vi "dis_on_test.vi"() -> ()   [LabVIEW 2011]
panel:
  in  "milliseconds to wait":u32=20
  in  "Starting Voltage":dbl=0.4
  in  "Goal Signal":dbl=1.0
  out "Generator Voltage 2":string
  out "Over 2":bool
  out "Signal 2":dbl
  out "Signal":dbl
  out "Over":bool
  out "Generator Voltage":string
  out "Read Back":string
  out "Check":string
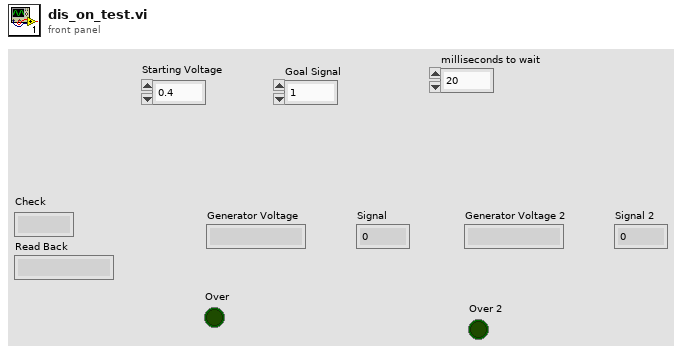
[diagram p1: front panel]
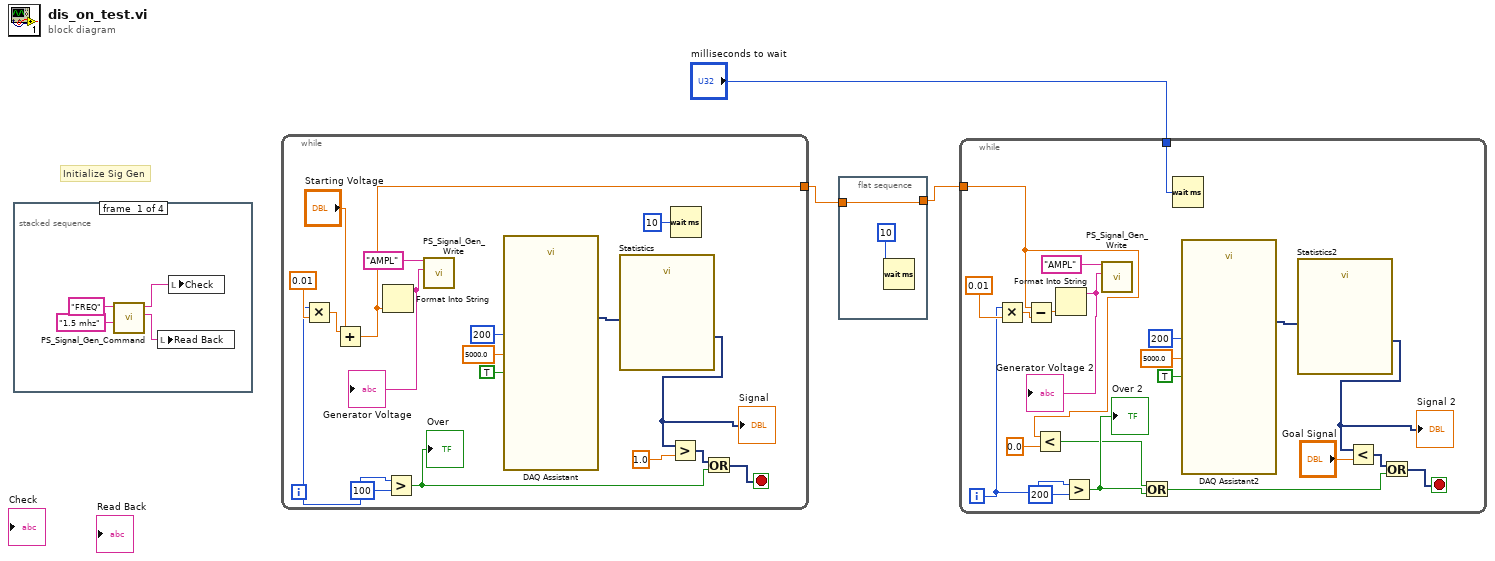
[diagram p0: block diagram]
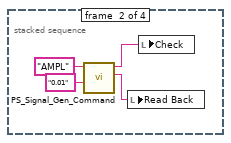
[diagram p2: hidden frame]
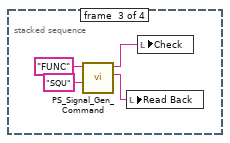
[diagram p3: hidden frame]
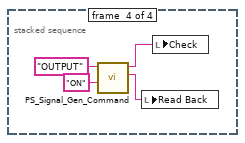
[diagram p4: hidden frame]
diagram:
  # "Initialize Sig Gen"
  n1 = stacked-sequence {
    frame #0 {
      n2 = call "PS_Signal_Gen_Command.vi"("Value String"="1.5 mhz", "Command String"="FREQ") -> ("Read Back"=w4:string, "Request String"=w5:string)  [unwired: 7 in, 1 out]
      n3 = local write "Read Back"(w4) -> ()
      n4 = local write "Check"(w5) -> ()
    }
    frame #1 {
      n5 = call "PS_Signal_Gen_Command.vi"("Value String"="0.01", "Command String"="AMPL") -> ("Read Back"=w8:string, "Request String"=w9:string)  [unwired: 7 in, 1 out]
      n6 = local write "Read Back"(w8) -> ()
      n7 = local write "Check"(w9) -> ()
    }
    frame #2 {
      n8 = call "PS_Signal_Gen_Command.vi"("Value String"="SQU", "Command String"="FUNC") -> ("Read Back"=w12:string, "Request String"=w13:string)  [unwired: 7 in, 1 out]
      n9 = local write "Read Back"(w12) -> ()
      n10 = local write "Check"(w13) -> ()
    }
    frame #3 {
      n11 = call "PS_Signal_Gen_Command.vi"("Value String"="ON", "Command String"="OUTPUT") -> ("Read Back"=w16:string, "Request String"=w17:string)  [unwired: 7 in, 1 out]
      n12 = local write "Read Back"(w16) -> ()
      n13 = local write "Check"(w17) -> ()
    }
  }
  n14 = while {
    tunnel: [w23] -> w3
    i -> [w36]
    stop <- w30 stop-if-true
    n15 = Multiply(x=w36, y=0.01) -> (x*y=w22:dbl)
    n16 = Add(x=w22, y="Starting Voltage") -> (x+y=w23:dbl)
    n17 = Format Into String(w23) -> (resulting string=w24:string)  [unwired: 3 in, 1 out]
    "Generator Voltage" <- w24
    n18 = Greater?(x=w36, y=100) -> (0:w26:bool)
    "Over" <- w26
    n19 = call "PS_Signal_Gen_Write.vi"("Value String"=w24, "Command String"="AMPL") -> ()  [unwired: 9 in, 1 out]
    n20 = call "DAQ Assistant"("rate"=5000.0, "number of samples"=200, "stop (F)"=TRUE) -> ("data"=w31:dynamicdata)  [unwired: 13 in, 3 out]
    n21 = call "Statistics"("Signals"=w31) -> ("Arithmetic Mean"=w25:dynamicdata)  [unwired: 24 in, 2 out]
    "Signal" <- w25
    n22 = Greater?(x=w25, y=1.0) -> (0:w28:dynamicdata)
    n23 = Wait (ms)(milliseconds to wait=u32 10) -> ()  [unwired: 1 out]
    n24 = Or(x=w28, y=w26) -> (x .or. y?=w30:dynamicdata)
  }
  n25 = flat-sequence {
    tunnel: [w38] -> w2
    tunnel: w3 -> [w38]
    frame #0 {
      n26 = Wait (ms)(milliseconds to wait=u32 10) -> ()  [unwired: 1 out]
    }
  }
  n27 = while {
    tunnel: w2 -> [w42]
    tunnel: "milliseconds to wait" -> [w40]
    i -> [w59]
    stop <- w53 stop-if-true
    n28 = Multiply(x=w59, y=0.01) -> (x*y=w48:dbl)
    n29 = Subtract(x=w42, y=w48) -> (x-y=w47:dbl)
    n30 = Less?(x=w42, y=0.0) -> (x < y?=w44:bool)
    n31 = Format Into String(w47) -> (resulting string=w50:string)  [unwired: 3 in, 1 out]
    "Generator Voltage 2" <- w50
    n32 = Greater?(x=w59, y=200) -> (0:w45:bool)
    "Over 2" <- w45
    n33 = call "PS_Signal_Gen_Write.vi"("Value String"=w50, "Command String"="AMPL") -> ()  [unwired: 9 in, 1 out]
    n34 = Or(x=w44, y=w45) -> (x .or. y?=w46:bool)
    n35 = Wait (ms)(milliseconds to wait=w40) -> ()  [unwired: 1 out]
    n36 = call "DAQ Assistant2"("rate"=5000.0, "number of samples"=200, "stop (F)"=TRUE) -> ("data"=w54:dynamicdata)  [unwired: 13 in, 3 out]
    n37 = call "Statistics2"("Signals"=w54) -> ("Arithmetic Mean"=w49:dynamicdata)  [unwired: 24 in, 2 out]
    "Signal 2" <- w49
    n38 = Less?(x=w49, y="Goal Signal") -> (x < y?=w52:dynamicdata)
    n39 = Or(x=w52, y=w46) -> (x .or. y?=w53:dynamicdata)
  }
